vi "绘制判定框.vi"(8 "error in (no error)":errorcluster caption="错误输入（无错误）", 10 "判定框类型":enum16{"区间", "终点"}(ring), 11 "曲线判定条件":T1) -> (0 "error out":errorcluster caption="错误输出", 3 "判定框":cluster{"横坐标":dbl[], "纵坐标":dbl[]}[](array[cluster]))   [LabVIEW 2019]
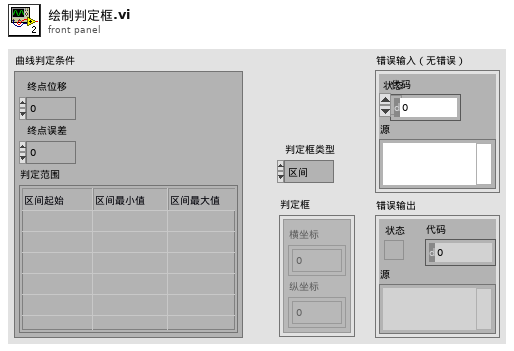
[diagram p1: front panel]
types:
  T1 = cluster{"终点位移":dbl, "终点误差":dbl, "判定范围":string[][]}
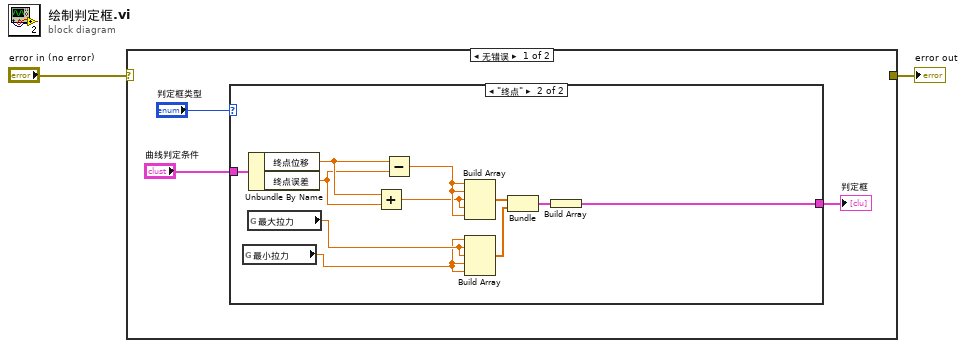
[diagram p0: block diagram]
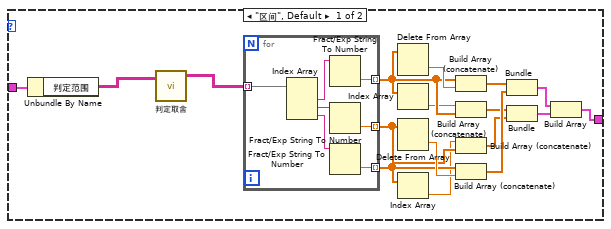
[diagram p2: hidden frame]
diagram:
  n1 = case shown="无错误" "error in (no error)" {
    selector: "error in (no error)" -> [_ w41]
    tunnel: [_ w41] -> w1
    frame No Error {
      n2 = case shown="\"终点\"" "判定框类型" {
        tunnel: "曲线判定条件" -> [w22 w40]
        tunnel: [w13 w32] -> w3
        frame "区间", Default {
          n3 = Unbundle By Name(w22) -> ("判定范围"=w21:string[][])
          n4 = call "判定取舍.vi"("判定 1"=w21) -> ("判定 3"=w20:string[][])  [unwired: 3 in]
          n5 = for {
            tunnel: w20 -> [w29] mode=indexing
            tunnel: [w27] -> w9 mode=indexing
            tunnel: [w24] -> w10 mode=indexing
            tunnel: [w23] -> w7 mode=indexing
            n6 = Index Array(array=w29) -> (element #1=w28:string, element #2=w26:string, element #3=w25:string)  [unwired: 3 in]
            n7 = Fract/Exp String To Number(string=w28) -> (number=w27:dbl)  [unwired: 3 in, 1 out]
            n8 = Fract/Exp String To Number(string=w26) -> (number=w23:dbl)  [unwired: 3 in, 1 out]
            n9 = Fract/Exp String To Number(string=w25) -> (number=w24:dbl)  [unwired: 3 in, 1 out]
          }
          n10 = Delete From Array(array=w9) -> (deleted portion=w15:dbl)  [unwired: 2 in, 1 out]
          n11 = Index Array(array=w9) -> (element=w8:dbl)  [unwired: 1 in]
          n12 = Delete From Array(array=w7) -> (deleted portion=w14:dbl)  [unwired: 2 in, 1 out]
          n13 = Index Array(array=w10) -> (element=w6:dbl)  [unwired: 1 in]
          n14 = Build Array (concatenate)(w9, w15) -> (w19:dbl[])
          n15 = Build Array (concatenate)(w8, w9) -> (w16:dbl[])
          n16 = Build Array (concatenate)(w6, w7) -> (w17:dbl[])
          n17 = Build Array (concatenate)(w10, w14) -> (w18:dbl[])
          n18 = Bundle(w19, w18) -> (w12:cluster{dbl[], dbl[]})  [unwired: 1 in]
          n19 = Bundle(w16, w17) -> (w11:cluster{dbl[], dbl[]})  [unwired: 1 in]
          n20 = Build Array(w12, w11) -> (w13:cluster{dbl[], dbl[]}[])
        }
        frame "终点" {
          n21 = global read "判定参数.vi" "最小拉力"() -> (w30:dbl)
          n22 = global read "判定参数.vi" "最大拉力"() -> (w31:dbl)
          n23 = Unbundle By Name(w40) -> ("终点位移"=w39:dbl, "终点误差"=w38:dbl)
          n24 = Add(x=w39, y=w38) -> (x+y=w36:dbl)
          n25 = Subtract(x=w39, y=w38) -> (x-y=w37:dbl)
          n26 = Build Array(w37, w37, w36, w36, w37) -> (w35:dbl[])
          n27 = Build Array(w30, w31, w31, w30, w30) -> (w34:dbl[])
          n28 = Bundle(w35, w34) -> (w33:cluster{dbl[], dbl[]})  [unwired: 1 in]
          n29 = Build Array(w33) -> (w32:cluster{dbl[], dbl[]}[])
        }
      }
      "判定框" <- w3
    }
    frame Error {
    }
  }
  "error out" <- w1
